vi "DriveDistanceX.vi"(2 "Parameter String":string, 3 "Reinit":bool) -> (0 "Error Out":errorcluster, 1 "Increment":bool)   [LabVIEW 2023]
doc: "The swerve drive base will translate in the field-centric X direction at a speed specified by the joystick command. This is a \"dumb\" algorithm, there is no feedback controller and the direction of translation must be specified manually. Any complex or critical translations should be handled using either the Path Follower or auto-targeting. \n\nParameters:\n1. relative travel distance in the field-centric X direction --> (in) [0,630]\n2. relative translation speed --> [-1,1]"
uses:
  SafeParser_Float.vi
  GlobalDriverStationCommands.vi
  GlobalPoseAndTargeting.vi
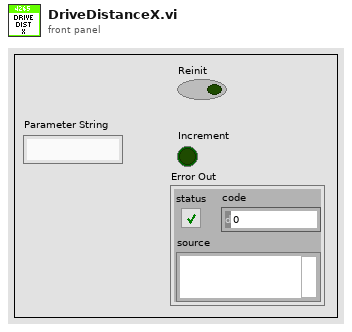
[diagram p1: front panel]
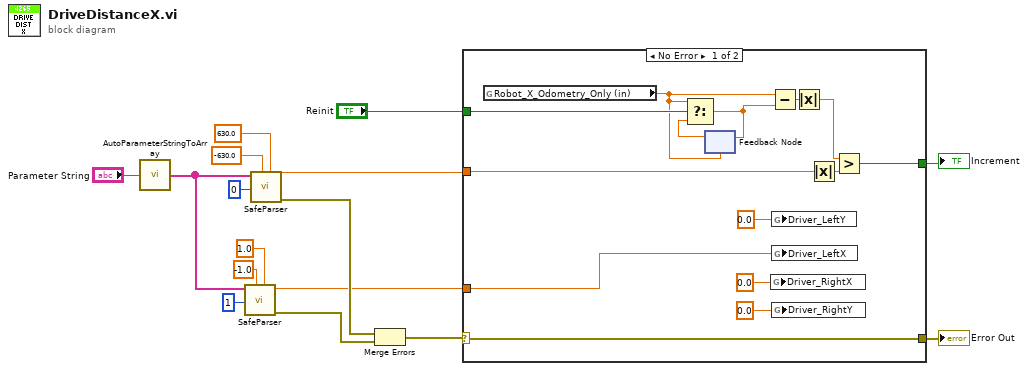
[diagram p0: block diagram]
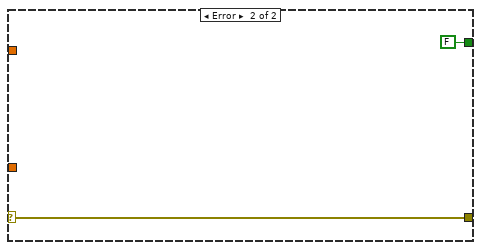
[diagram p2: hidden frame]
diagram:
  n1 = call "AutoParameterStringToArray.vi"("Parameter String"="Parameter String") -> ("Parsed Parameters"=w9:string[])
  n2 = call-poly "SafeParser.vi"("Maximum"=1.0, "Minimum"=-1.0, "Array Index"=1 ("Parameter Index"), "String Array"=w9) -> ("Error Out"=w7:errorcluster, "Typecast  Value"=w4:dbl)  [unwired: 6 in]
  n3 = call-poly "SafeParser.vi"("Maximum"=630.0, "Minimum"=-630.0, "Array Index"=0 ("Parameter Index"), "String Array"=w9) -> ("Error Out"=w6:errorcluster, "Typecast  Value"=w8:dbl)  [unwired: 6 in]
  n4 = Merge Errors(w6, w7) -> (w5:errorcluster)
  n5 = case shown="No Error" w5 {
    selector: w5 -> [w20 w32]
    tunnel: [w30 FALSE] -> w1
    tunnel: "Reinit" -> [w28 _]
    tunnel: [w20 w32] -> w15
    tunnel: w8 -> [w19 _]
    tunnel: w4 -> [w18 _]
    frame No Error {
      n6 = global read "GlobalPoseAndTargeting.vi" "Robot_X_Odometry_Only (in)"() -> (w27:dbl)
      n7 = feedback #1(w27) -> (w29:dbl)
      n8 = Select(t=w27, s=w28, f=w29) -> (s? t:f=w26:dbl)
      n9 = feedback-in #1(w26) -> ()
      n10 = Subtract(x=w27, y=w26) -> (x-y=w25:dbl)
      n11 = global write "GlobalDriverStationCommands.vi" "Driver_RightX"(0.0 ("Driver_RightX")) -> ()
      n12 = global write "GlobalDriverStationCommands.vi" "Driver_LeftY"(0.0 ("Driver_LeftY")) -> ()
      n13 = global write "GlobalDriverStationCommands.vi" "Driver_LeftX"(w18) -> ()
      n14 = global write "GlobalDriverStationCommands.vi" "Driver_RightY"(0.0 ("Driver_RightX")) -> ()
      n15 = Absolute Value(x=w25) -> (abs(x)=w22:dbl)
      n16 = Absolute Value(x=w19) -> (abs(x)=w21:dbl)
      n17 = Greater?(x=w22, y=w21) -> (0:w30:bool)
    }
    frame Error {
    }
  }
  "Increment" <- w1
  "Error Out" <- w15
